vi "MacroOpsManager_MD_old.vi"() -> ()   [LabVIEW 2012]
doc: "SciScan 1.2 160622"
uses:
  SubVIs/Timer_MacroInterpreter_Commands.ctl
  GFG/GFG library.lvlib
panel:
  out "number 3":dbl
  out "number 2":dbl
  out "number":dbl
  in  "stop":bool
  out "Error Out":errorcluster
  in  "Error In":errorcluster
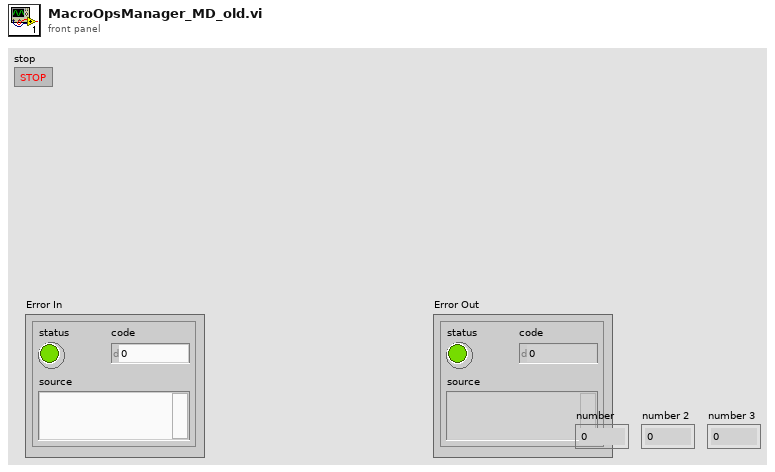
[diagram p1: front panel]
types:
  T1 = typedef "Timer_MacroInterpreter_Commands.ctl" = enum16{"Start", "Pause", "Run"}
  T2 = cluster{"moveXabs":dbl, "moveYabs":dbl, "moveZabs":dbl}
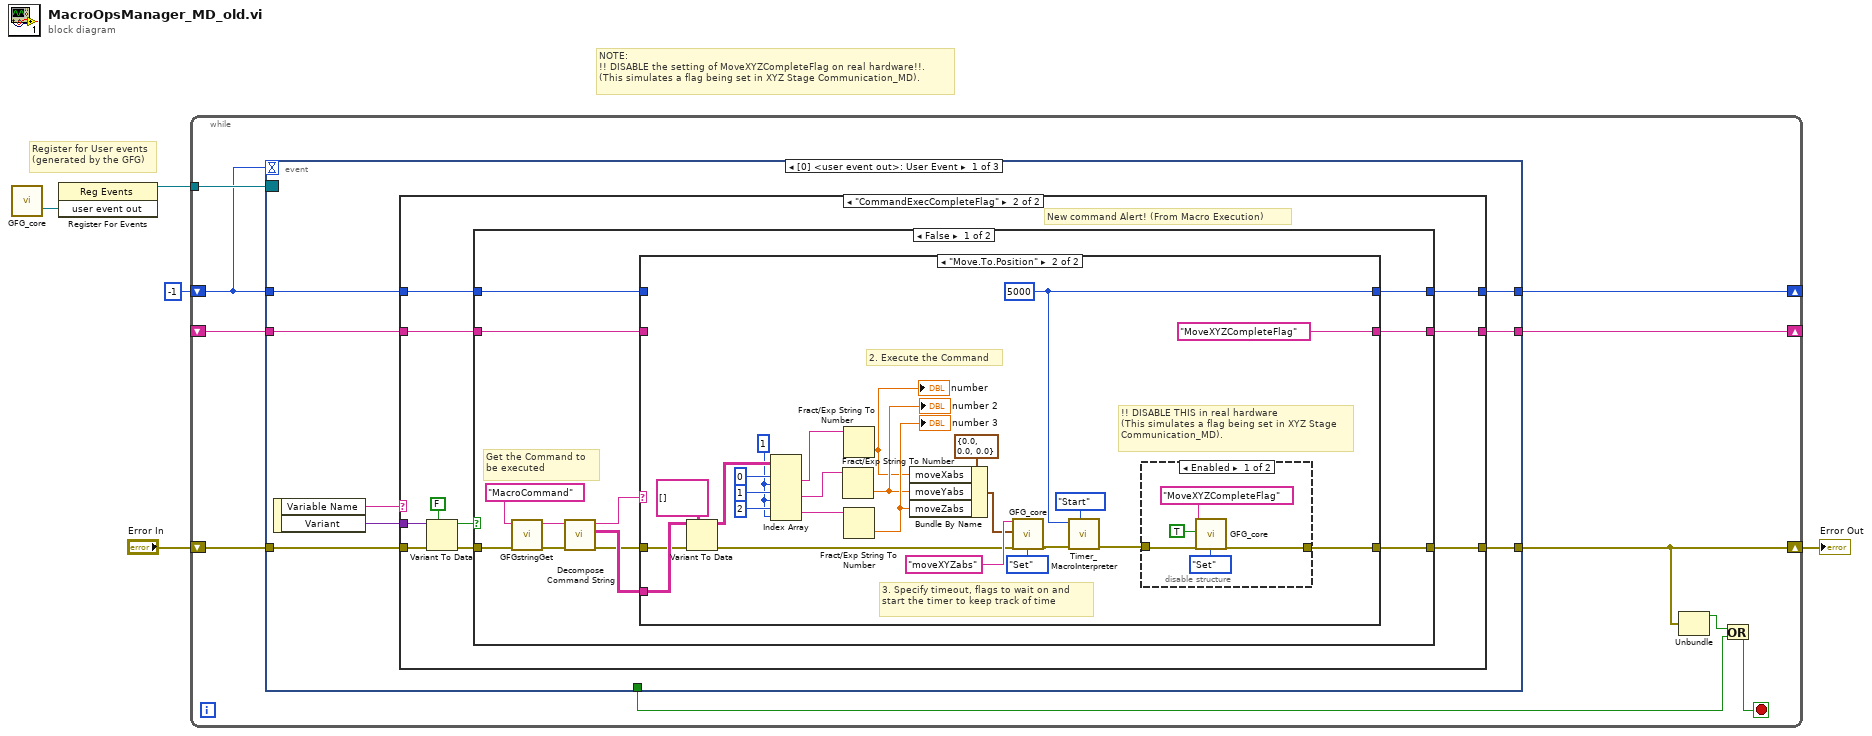
[diagram p0: block diagram]
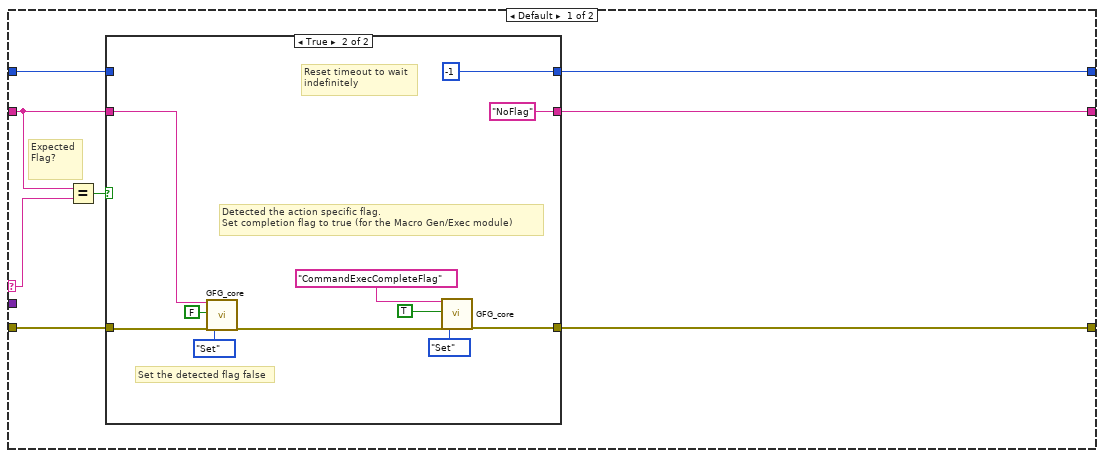
[diagram p2: hidden frame]
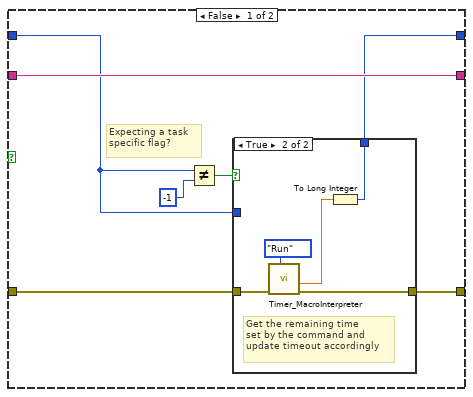
[diagram p3: hidden frame]
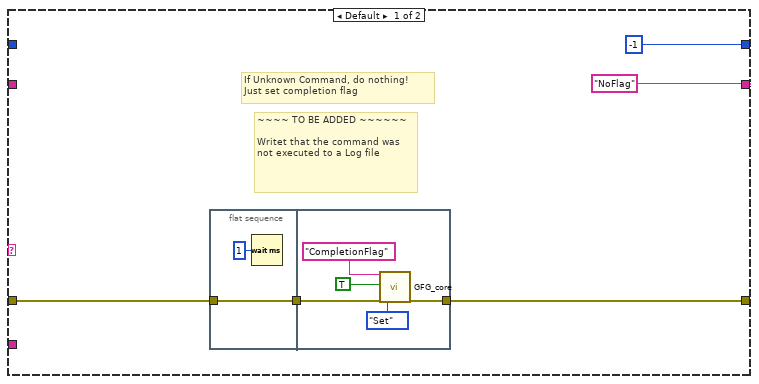
[diagram p5: hidden frame]
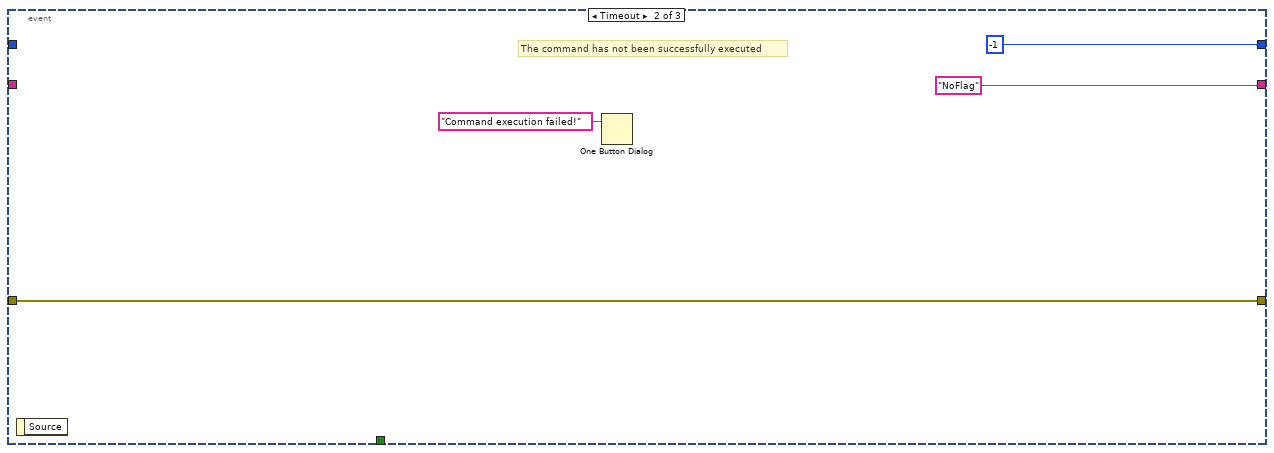
[diagram p8: hidden frame]
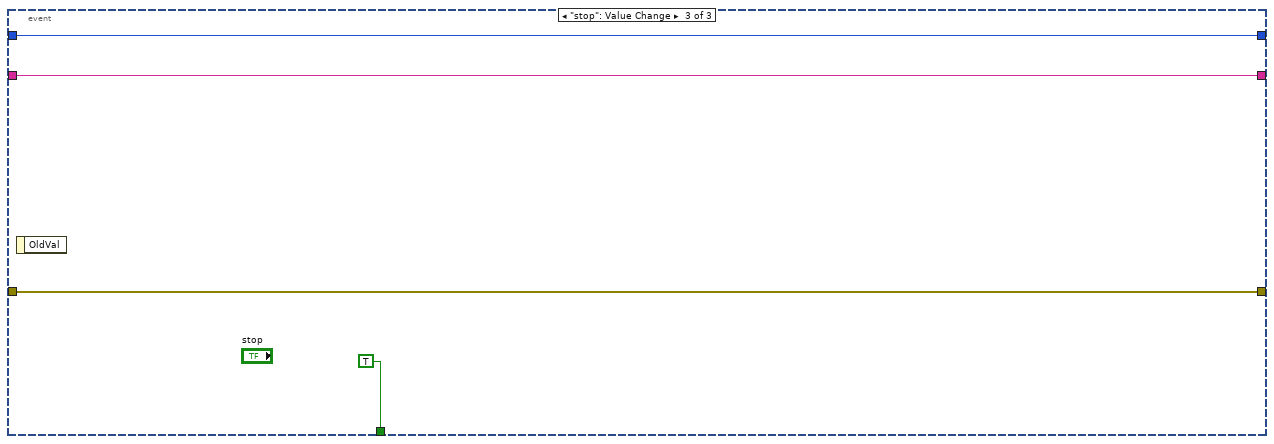
[diagram p9: hidden frame]
diagram:
  # "NOTE:\n!! DISABLE the setting of MoveXYZCompleteFlag on real hardware!!.\n(This simulates a flag being set in XYZ Stage Communication_MD)."
  # "Register for User events\n(generated by the GFG)"
  n1 = call "GFG_core.vi"() -> ("user event out"=w5:refnum<user-event>)  [unwired: 13 in, 6 out]
  n2 = register-events(w5) -> (reference out=w4:refnum<event-registration>)  [unwired: 2 in, 1 out]
  n3 = while {
    tunnel: w4 -> [w15]
    shift-right: [w13] -> _
    shift-left: _ -> [w12]
    shift-right: [w11] -> _
    shift-left: -1 -> [w10]
    shift-right: [w9] -> w1
    shift-left: "Error In" -> [w14]
    stop <- w6 stop-if-true
    n4 = event shown="[0] <user event out>: User Event" {
      selector: w15 -> [_ _ _]
      dyn-events: _ -> [_ _ _]
      timeout: w10 -> [_ _ _]
      tunnel: w14 -> [w22 w124 w127]
      tunnel: [_ _ TRUE] -> w7
      tunnel: [w20 "NoFlag" ("Variable Name in") w129] -> w13
      tunnel: w12 -> [w17 _ w129]
      tunnel: [w19 -1 w128] -> w11
      tunnel: w10 -> [w18 _ w128]
      tunnel: [w16 w124 w127] -> w9
      event User Event {
        n5 = event-data() -> ("Variable Name"=w23:string, "Variant"=w21:variant)  [unwired: 1 in]
        n6 = case shown="\"CommandExecCompleteFlag\"" w23 {
          selector: w23 -> [w31 _]
          tunnel: w22 -> [w24 w64]
          tunnel: w21 -> [_ w65]
          tunnel: [w27 w61] -> w20
          tunnel: [w29 w60] -> w19
          tunnel: w18 -> [w30 w59]
          tunnel: w17 -> [w28 w58]
          tunnel: [w26 w57] -> w16
          frame Default {
            # "Expected Flag?"
            n7 = Equal?(x=w28, y=w31) -> (x = y?=w25:bool)
            n8 = case shown="True" w25 {
              tunnel: w30 -> [w32 _]
              tunnel: [w33 -1] -> w29
              tunnel: [w38 "NoFlag" ("Variable Name in")] -> w27
              tunnel: w28 -> [w38 w47]
              tunnel: w24 -> [w35 w48]
              tunnel: [w34 w51] -> w26
              frame False {
                # "Expecting a task specific flag?"
                n9 = Not Equal?(x=w32, y=-1) -> (x != y?=w36:bool)
                n10 = case shown="True" w36 {
                  tunnel: w35 -> [w39 w44]
                  tunnel: [w39 w42] -> w34
                  tunnel: [w40 w41] -> w33
                  tunnel: w32 -> [w40 _]
                  frame False {
                    # "Wait indefinitely\n(timeout = -1)"
                  }
                  frame True {
                    # "Get the remaining time\nset by the command and\nupdate timeout accordingly"
                    n11 = call "Timer_MacroInterpreter.vi"("Timer Command"=Timer_MacroInterpreter_Commands."Run", "Error In"=w44) -> ("Error Out"=w42:errorcluster, "Remaining Time (ms)"=w43:dbl)  [unwired: 6 in, 2 out]
                    n12 = To Long Integer(number=w43) -> (32bit integer=w41:i32)
                  }
                }
              }
              frame True {
                # "Reset timeout to wait\nindefinitely"
                # "Set the detected flag false"
                # "Detected the action specific flag.\nSet completion flag to true (for the Macro Gen/Exec module)"
                n13 = call "GFG_core.vi"("Variable Name in"=w47, "Variant in"=FALSE, "error in (no error)"=w48, "Action"=enum16{"Init", "Set", "Get", "Clear"}."Set") -> ("error out"=w46:errorcluster)  [unwired: 9 in, 6 out]
                n14 = call "GFG_core.vi"("Variable Name in"="CommandExecCompleteFlag", "Variant in"=TRUE, "error in (no error)"=w46, "Action"=enum16{"Init", "Set", "Get", "Clear"}."Set") -> ("error out"=w51:errorcluster)  [unwired: 9 in, 6 out]
              }
            }
          }
          frame "CommandExecCompleteFlag" {
            # "New command Alert! (From Macro Execution)"
            n15 = Variant To Data(error in=w64, type=FALSE, Variant=w65) -> (data=w63:bool, error out=w62:errorcluster)
            n16 = case shown="False" w63 {
              tunnel: w62 -> [w72 w120]
              tunnel: [w71 w121] -> w61
              tunnel: [w70 w122] -> w60
              tunnel: w59 -> [w68 w122]
              tunnel: w58 -> [w69 w121]
              tunnel: [w67 w120] -> w57
              frame False {
                # "Get the Command to\nbe executed"
                n17 = call "GFGstringGet.vi"("Variable Name in"="MacroCommand" ("Source VI")) -> ("String"=w75:string)  [unwired: 9 in, 1 out]
                n18 = call "Decompose Command String.vi"("Error In"=w72, "Command IN"=w75) -> ("Error Out"=w73:errorcluster, "Parameter Table"=w74:string[][], "Action"=w77:string)  [unwired: 6 in, 1 out]
                n19 = case shown="\"Move.To.Position\"" w77 {
                  tunnel: w74 -> [_ w97]
                  tunnel: w73 -> [w81 w92]
                  tunnel: ["NoFlag" ("Variable Name in") "MoveXYZCompleteFlag" ("Variable Name in")] -> w71
                  tunnel: [-1 w94] -> w70
                  tunnel: w69 -> [_ _]
                  tunnel: w68 -> [_ _]
                  tunnel: [w78 w90] -> w67
                  frame Default {
                    # "~~~~ TO BE ADDED ~~~~~~\n\nWritet that the command was not executed to a Log file"
                    # "If Unknown Command, do nothing!\nJust set completion flag"
                    n20 = flat-sequence {
                      tunnel: [w83] -> w82
                      tunnel: w81 -> [w83]
                      tunnel: w82 -> [w86]
                      tunnel: [w85] -> w78
                      frame #0 {
                        n21 = Wait (ms)(milliseconds to wait=u32 1) -> ()  [unwired: 1 out]
                      }
                      frame #1 {
                        n22 = call "GFG_core.vi"("Variable Name in"="CompletionFlag", "Variant in"=TRUE, "error in (no error)"=w86, "Action"=enum16{"Init", "Set", "Get", "Clear"}."Set") -> ("error out"=w85:errorcluster)  [unwired: 9 in, 6 out]
                      }
                    }
                  }
                  frame "Move.To.Position" {
                    w94 = 5000
                    w109 = 1 ("disabled index (col)")
                    # "!! DISABLE THIS in real hardware\n(This simulates a flag being set in XYZ Stage\nCommunication_MD)."
                    # "3. Specify timeout, flags to wait on and start the timer to keep track of time"
                    # "2. Execute the Command"
                    n23 = Variant To Data(error in=w92, type=string[][] [], Variant=w97) -> (data=w113:string[][], error out=w101:errorcluster)
                    n24 = Index Array(array=w113, index (row) #1=0 ("disabled index (row)"), index (col) #1=w109, index (row) #2=1 ("disabled index (row)"), index (col) #2=w109, index (row) #3=2 ("disabled index (row)"), index (col) #3=w109) -> (element #1=w108:string, element #2=w107:string, element #3=w106:string)
                    n25 = Fract/Exp String To Number(string=w107) -> (number=w99:dbl)  [unwired: 3 in, 1 out]
                    "number 2" <- w99
                    n26 = Fract/Exp String To Number(string=w108) -> (number=w98:dbl)  [unwired: 3 in, 1 out]
                    "number" <- w98
                    n27 = Fract/Exp String To Number(string=w106) -> (number=w100:dbl)  [unwired: 3 in, 1 out]
                    "number 3" <- w100
                    n28 = Bundle By Name(cluster=T2 {"moveXabs"=0.0, "moveYabs"=0.0, "moveZabs"=0.0} ("output cluster"), "moveXabs"=w98, "moveYabs"=w99, "moveZabs"=w100) -> (w102:T2)
                    n29 = call "GFG_core.vi"("Variable Name in"="moveXYZabs", "Variant in"=w102, "error in (no error)"=w101, "Action"=enum16{"Init", "Set", "Get"}."Set") -> ("error out"=w93:errorcluster)  [unwired: 9 in, 6 out]
                    n30 = call "Timer_MacroInterpreter.vi"("Timer Command"=Timer_MacroInterpreter_Commands."Start", "Error In"=w93, "Set Time (ms)"=w94) -> ("Error Out"=w91:errorcluster)  [unwired: 5 in, 3 out]
                    n31 = disable-structure shown="Enabled" {
                      disable-tunnel: w91 -> [w119 _]
                      disable-tunnel: [w118 _] -> w90
                      frame Enabled {
                        n32 = call "GFG_core.vi"("Variable Name in"="MoveXYZCompleteFlag", "Variant in"=TRUE, "error in (no error)"=w119, "Action"=enum16{"Init", "Set", "Get"}."Set") -> ("error out"=w118:errorcluster)  [unwired: 9 in, 6 out]
                      }
                      frame Disabled {
                      }
                    }
                  }
                }
              }
              frame True {
                # "UNexpected value!  (Expecting a FALSE for the \"CompletionFlag\").\n -- Do nothing --"
              }
            }
          }
        }
      }
      event Timeout {
        # "The command has not been successfully executed"
        n33 = event-data() -> ()  [unwired: 1 in, 1 out]
        n34 = One Button Dialog(message="Command execution failed!") -> ()  [unwired: 1 in, 1 out]
      }
      event "stop": Value Change {
        n35 = event-data() -> ()  [unwired: 1 in, 1 out]
      }
    }
    n36 = Unbundle(w9) -> ("status"=w8:bool)  [unwired: 2 out]
    n37 = Or(x=w8, y=w7) -> (x .or. y?=w6:bool)
  }
  "Error Out" <- w1
